vi "EnFlo_Tunnel_Setup.vi"() -> ()   [LabVIEW 2020]
uses:
  ADAM Controls/Update_scan_value.ctl
  ADAM Controls/Module_type_ADAM.ctl
  ADAM Controls/Function_ADAM.ctl
  ADAM Controls/Channel_State.ctl
  ADAM Controls/Calib_type_ADAM.ctl
  ADAM Controls/Address.ctl
  ADAM Controls/Ch_description_ADAM.ctl
panel:
  in  "Desired Lab Air Temp":dbl format="%.2f"
  out "Numerical Values":dbl[](array[numeric]) format="%.9f"
  out "Ch Description Array":T1[](array[typedef]) {"Duty" format="%016b"; "D" format="%#_5g"; "C" format="%#_5g"; "B" format="%#_5g"; "A" format="%#_5g"}
  in  "Traverse Origin X Offset (mm)":dbl min=0.0 max=20000.0
  in  "Show Heater Setup":bool
  in  "stop":bool
  in  "Desired Chilled Water Temp":dbl format="%.2f"
  out "Reference Anemometer":string
  in  "OK":bool
  in  "Wind Direction (Deg)":dbl format="%.2f"
  in  "Obstacle/Building":u16(ring) items=["1-500 DAPPLE low Res", "100mm Trench", "100x100 Cube", "100x100 pressure tapped cube", "100x100x200 Tall", "100x100x300 Tall", "100x100x400mm Tall", "110mm cube array 110mm spacing", "110mm cube array 55mm spacing", "12 WTs", "150*150*150mm cube", "16 blocks 55 x 55 x 110mm tall centre at x=12m", "16 buildings 250*500*125mm", "16 x 110mm cube array 110mm spacing", "20 buildings 500x250x125mm", "25 x 110mm cube array 110mm spacing", "25mm Trench in 1.4m Turntable", "4 buildings 750x500x125mm", "4 x 110mm cube array 110mm spacing", "400mm x 400mm Heated Mat centre 12m", "500x250x125 Block", "500x300mm Trees 100mm tall", "660mm x 3000mm Heated Mat centre 12m", "70x140x70bldgs 12x19rows 1x3h Building", "70x140x70bldgs 14x21row", "70x140x70bldgs 14x29 row", "9 x 110mm cube array 110mm spacing", "990mm x 3000mm Heated Mat centre 14m", "Array of 24 tanks dia 130mm height 88mm", "Blade 1", "Blade 2", "Building With Single Stack", "Building with Twin Stack", "Champs Elysees Source 1", "Champs Elysees Source 2", "Champs Elysees Source 3", "Complex - All buildings", "Complex - only 2 buildings", "Complex Array", "Concawe Actual Model 6 Cylinders", "DAPPLE Dome Centre", "DAPPLE Dome Centre with station", "DAPPLE high Res buildings at intersection", "DAPPLE low Res", "DAPPLE low Res with roof roughness", "DAPPLE low Res(model+B42-45 and obstacles in the west of the model)", "DAPPLE low Res(sampling at Mary  Rd  Model+B42-45)", "DAPPLE low Res(sampling at Mary  Rd with B38-41and A5)", "DAPPLE low Res(sampling at Mary  Rd without B38-41)", "DAPPLE low Res(sampling at Mary. Rd add A1-5)", "DYCE_London_110mm", "False Floor (table 4.17m x 0.9m  height 230mm)", "Forest at x=11003", "Group of 2 Tanks D=133mm upstream tank", "Group of 6 Tanks D=400mm no downstream tanks", "Group of 9 Tanks D=133mm Centre releasing 67mm roof heights", "Group of 9 Tanks D=400mm 3 downstream tanks", "HRModUrb SimpleC", "HRModUrb SimpleC with tall building", "HRModUrb SimpleV", "Headstart07 building", "Mesh Wool Disc Trees 220mm spacing", "Moditic_Bump", "Moditic_Bump_0-1385mm_200mm false floor", "Moditic_Bump_0-1385mm_200mm false floor No roughness", "Moditic_Bump_0-1385mm_200mm false floor with Array", "Moditic_Bump_0-1385mm_200mm false floor with Array_2", "Network Regular", "None", "Norway 1:300", "Norway 1:500", "ROSE (Bremen)", "Row_of_blocks_H=204_L=250mm", "S1_0Deg", "S1_45Deg", "S2_0Deg", "Sellafiield Site Model", "Sellafiield Site Model (Flat)", "Single Turbine II", "Single wind turbine (blade II) at X=10000 Y=0", "St Thomas Hospital - East Wing - Unclad", "St Thomas Hospital - East Wing - clad", "Storage Tank H=100  D=400mm", "Storage Tank H=100  D=400mm with 0 Deg Bund", "Storage Tank H=100  D=400mm with 45 Deg Bund", "Storage Tank H=100  D=400mm with Bund plus upstream tank", "Storage Tank H=100 D=500mmStorage Tank H=100  D=700mm", "Storage Tank H=89  D=133mm", "Storage Tank H=89  D=133mm with 0 Deg Bund", "Storage Tank H=89  D=133mm with 266mm Bund on turn table", "Storage Tank H=89  D=133mm with 45 Deg Bund", "Subfloor trench 285x285x3m", "Tree 171 mm - Dense", "Tree 171 mm - Porous", "Tree 91 mm - Dense", "Tree 91 mm - Porous", "Tree85mmRow - x=13000", "Two-Buildings Config", "Vehicle 1to20 - False Floor (table 4.17m x 0.9m  height 230mm)", "Vehicle 1to5 - False Floor (table 4.17m x 0.9m  height 230mm)", "WT Array1", "WT Array2", "WT Array21", "WT Array3", "WT Array4", "WT Array5", "WT Array6", "WT Array7", "WT x 2", "WT x 3", "WT x 4", "Edit Strings"]
  in  "Vorticity Generators":u16(ring) items=["5 Irwin spires 1.26m   X=50mm Y spacing 630mm", "5 Irwin spires 1.2m   X=50mm Y spacing 700mm", "Not Installed", "Offshore 13x TruncIrwin (H:600)  B(H:0):60  B(H:600):4  Yspace: 266  X:3925", "Offshore 13x TruncIrwin (H:600)  B(H:0):60  B(H:600):4  Yspace: 266  X:50", "Offshore 21x TruncIrwin (H:600)  B(H:0):60  B(H:600):4  Yspace: 167  X:50", "Offshore 5x TruncIrwin (H:1490)  B(H:0):150  B(H:1490):10  Yspace:660  X:50", "Offshore 5x TruncIrwin (H:1490)  B(H:0):150  B(H:700):10  Yspace:660  X:50", "Offshore 5x TruncIrwin (H:300)  B(H:0):150  B(H:300):10  Yspace:660  X:50", "Offshore 5x TruncIrwin (H:300)  B(H:0):30  B(H:300):2  Yspace:132  X:50", "Offshore 8x TruncIrwin (H:300)  B(H:0):150  B(H:300):10  Yspace:420  X:50", "Onshore 5xTruncNonIrwin (H:1490  B(H:0-120):250  B(H:192):177  B(H:1490):24)  YSpace:660 X:50", "Edit Strings"]
  in  "Side Wall Separation":u16(ring) items=["1.07m", "1.5m", "2.0m", "2.5m", "2.93m", "3m  from x=0.67 to x=10.67m", "3m  from x=0.67 to x=12.67m", "3m  from x=0.67 to x=18m", "3m  from x=0.67 to x=6.67m", "3m  from x=12 to x=18m", "3m  from x=2 to x=19m", "3m  from x=8 to x=18m", "No sidewalls installed", "Edit Strings"]
  in  "Roughness Height":u16(ring) items=["H=16mm  W=50mm Yspace=510mm Xspace=360mm Staggered", "H=20mm W=80mm YSpace=240mm  XSpace=240mm Staggered", "H=20mm W=80mm YSpace=240mm  XSpace=720mm Staggered", "no roughness elements (smooth)", "Edit Strings"]
  # "Boundary Layer Generation setup"
  # "This value should be zero if working in tunnel coordinates  (X=0 at start of working section)"
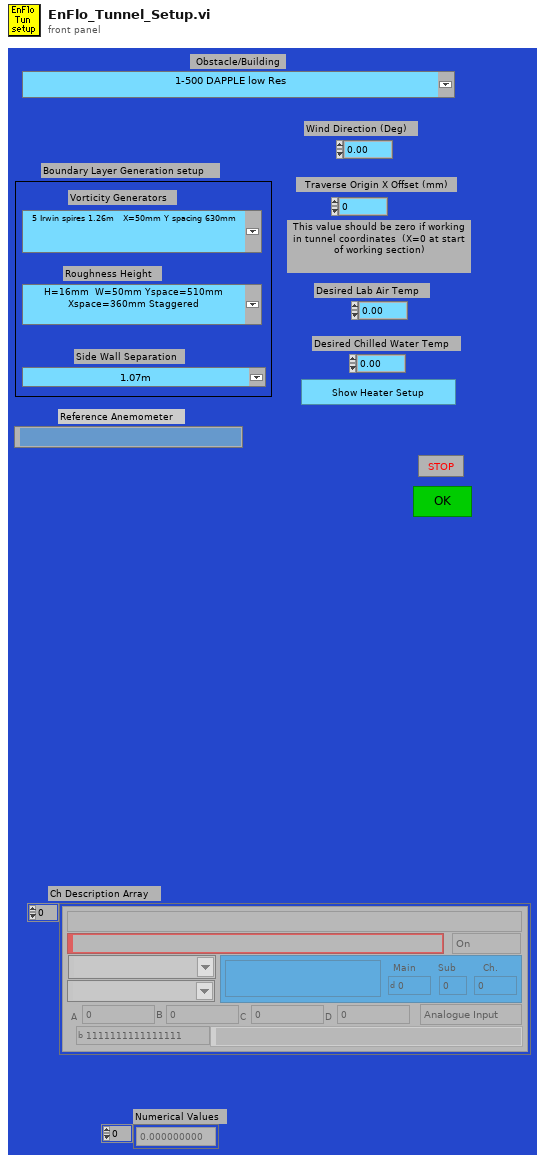
[diagram p1: front panel]
types:
  T1 = typedef "Ch_description_ADAM.ctl" = cluster{"Ch Name":string, "Type":T2, "Function":T3, "Ch State":T4, "Calibration type":T5, "A":dbl, "B":dbl, "C":dbl, "D":dbl, "Comments":string, "Address":T6, "String":string, "Duty":u16}
  T2 = typedef "Module_type_ADAM.ctl" = string
  T3 = typedef "Function_ADAM.ctl" = enum16{"Analogue Input", "Digital Input", "Event counter", "Event rate", "Analogue Output", "Digital Output", "Relay Output"}
  T4 = typedef "Channel_State.ctl" = enum16{"On", "Off", "Always On", "Always Off"}
  T5 = typedef "Calib_type_ADAM.ctl" = string
  T6 = typedef "Address.ctl" = cluster{"Main":i32, "Ch.":i32, "Sub":i32, "Port Name":string}
  T7 = typedef "Update_scan_value.ctl" = cluster{"Channel Name":string, "New Value":dbl}
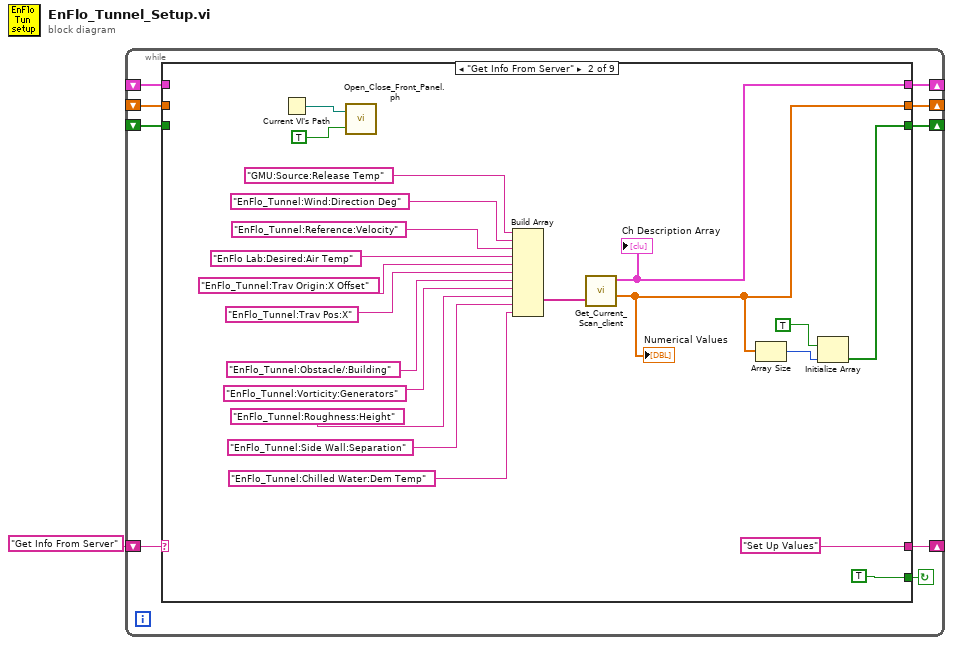
[diagram p0: block diagram]
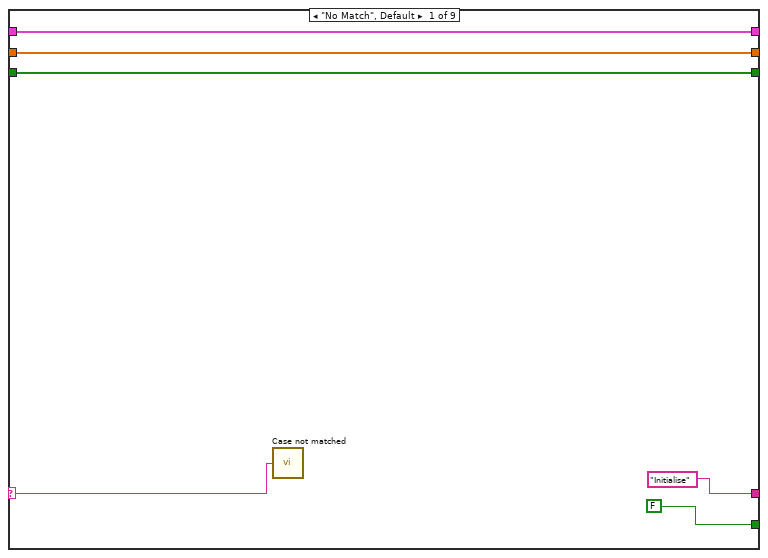
[diagram p2: hidden frame]
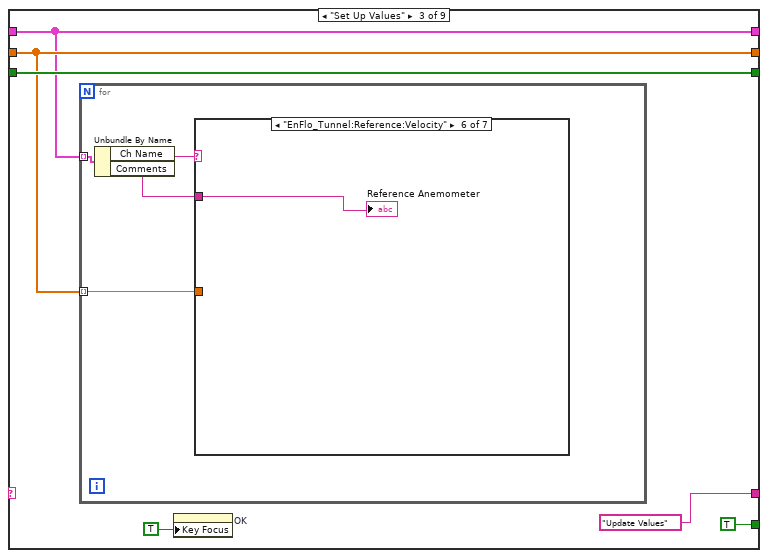
[diagram p3: hidden frame]
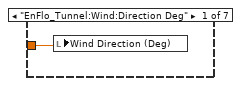
[diagram p4: hidden frame]
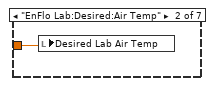
[diagram p5: hidden frame]
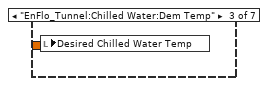
[diagram p6: hidden frame]
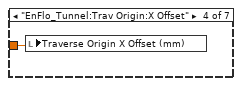
[diagram p7: hidden frame]
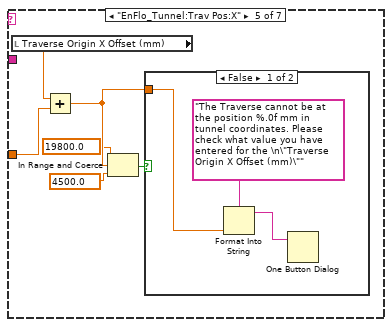
[diagram p8: hidden frame]
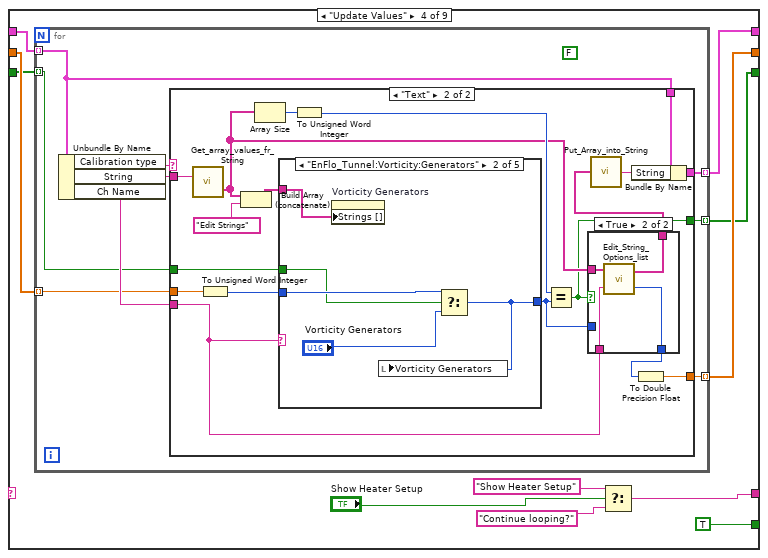
[diagram p11: hidden frame]
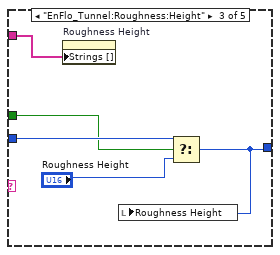
[diagram p15: hidden frame]
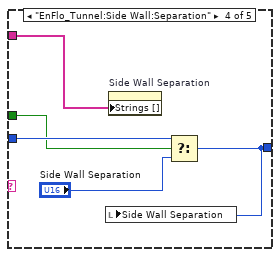
[diagram p16: hidden frame]
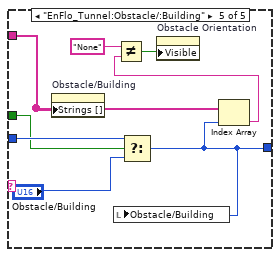
[diagram p17: hidden frame]
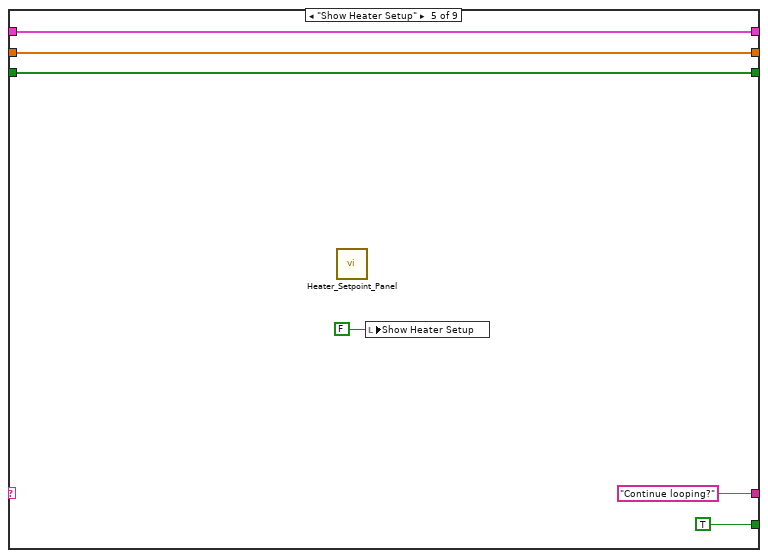
[diagram p18: hidden frame]
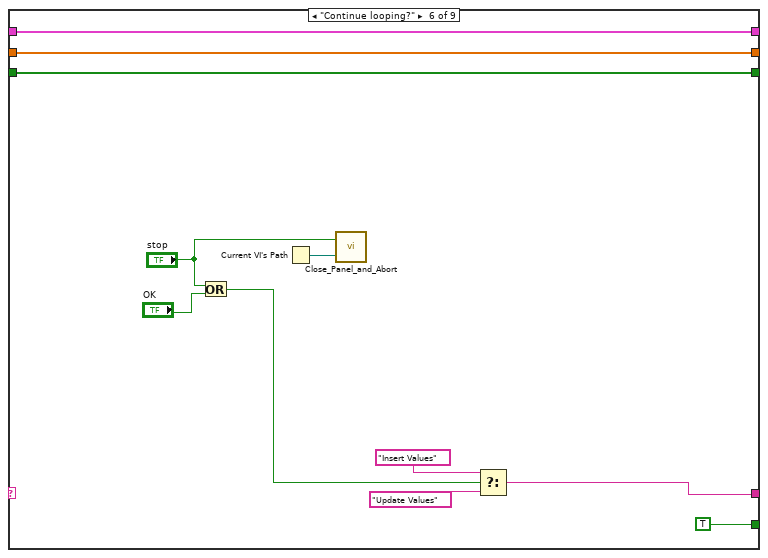
[diagram p19: hidden frame]
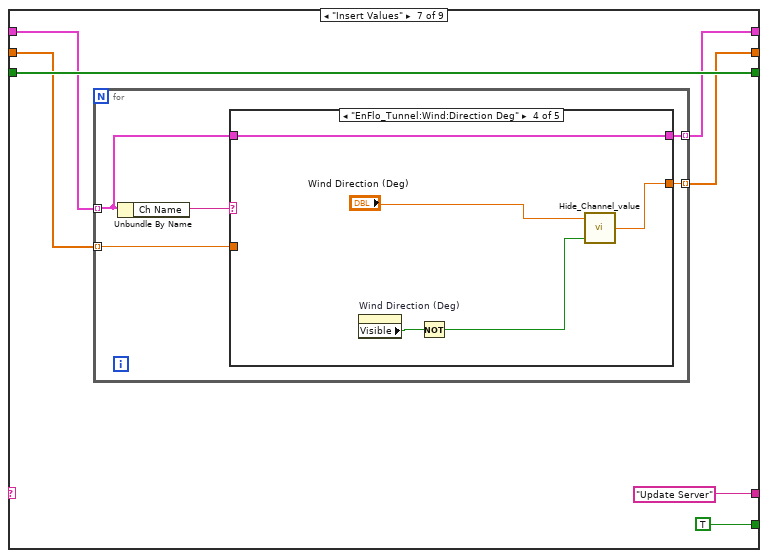
[diagram p20: hidden frame]
diagram:
  n1 = while {
    shift-left: _ -> [w2]
    shift-right: [w3] -> _
    shift-left: _ -> [w4]
    shift-right: [w6] -> _
    shift-left: _ -> [w5]
    shift-right: [w7] -> _
    shift-left: "Get Info From Server" -> [w8]
    shift-right: [w9] -> _
    stop <- w10 continue-if-true
    n2 = case shown="\"Get Info From Server\"" w8 {
      selector: w8 -> [w11 _ _ _ _ _ _ _ _]
      tunnel: [FALSE TRUE TRUE ("T button?") TRUE ("T button?") TRUE ("T button?") TRUE ("T button?") TRUE ("T button?") TRUE ("T button?") FALSE ("T button?")] -> w10
      tunnel: ["Initialise" "Set Up Values" "Update Values" w66 "Continue looping?" w140 "Update Server" "Add comments etc" "End"] -> w9
      tunnel: [w14 w28 w39 w70 w138 w149 w150 w182 w226] -> w7
      tunnel: [w13 w27 w40 w68 w137 w148 w153 w181 w225] -> w6
      tunnel: w5 -> [w14 _ w39 w71 w138 w149 w151 w182 w226]
      tunnel: w4 -> [w13 _ w40 w69 w137 w148 w152 w181 w225]
      tunnel: [w12 w24 w42 w62 w134 w146 w155 w180 w223] -> w3
      tunnel: w2 -> [w12 _ w42 w63 w134 w146 w155 w180 w223]
      frame "No Match", Default {
        n3 = call "Case not matched.vi"("Case Name not Matched"=w11) -> ()
      }
      frame "Get Info From Server" {
        n4 = Current VI's Path() -> (path=w22:path)
        n5 = call "Open_Close_Front_Panel.ph.vi"("Front Panel Window:Open"=TRUE, "VI path"=w22) -> ()  [unwired: 2 out]
        n6 = Build Array("GMU:Source:Release Temp", "EnFlo_Tunnel:Wind:Direction Deg", "EnFlo_Tunnel:Reference:Velocity", "EnFlo Lab:Desired:Air Temp", "EnFlo_Tunnel:Trav Origin:X Offset", "EnFlo_Tunnel:Trav Pos:X", "EnFlo_Tunnel:Obstacle/:Building", "EnFlo_Tunnel:Vorticity:Generators", "EnFlo_Tunnel:Roughness:Height", "EnFlo_Tunnel:Side Wall:Separation", "EnFlo_Tunnel:Chilled Water:Dem Temp") -> (w35:string[])
        n7 = call "Get_Current_Scan_client.vi"("multipleChannels"=w35) -> ("Ch Description Array"=w28:T1[], "Numerical Values"=w27:dbl[])  [unwired: 2 in, 1 out]
        "Ch Description Array" <- w28
        "Numerical Values" <- w27
        n8 = Array Size(array=w27) -> (size(s)=w26:i32)
        n9 = Initialize Array(TRUE, w26) -> (w24:bool[])
      }
      frame "Set Up Values" {
        n10 = for {
          tunnel: w40 -> [w47] mode=indexing
          tunnel: w39 -> [w46] mode=indexing
          n11 = Unbundle By Name(w46) -> ("Ch Name"=w45:string, "Comments"=w44:string)
          n12 = case shown="\"EnFlo_Tunnel:Reference:Velocity\"" w45 {
            tunnel: w47 -> [w48 w49 w50 w51 w56 _ _]
            tunnel: w44 -> [_ _ _ _ _ w61 _]
            frame "EnFlo_Tunnel:Wind:Direction Deg" {
              n13 = local write "Wind Direction (Deg)"(w48) -> ()
            }
            frame "EnFlo Lab:Desired:Air Temp" {
              n14 = local write "Desired Lab Air Temp"(w49) -> ()
            }
            frame "EnFlo_Tunnel:Chilled Water:Dem Temp" {
              n15 = local write "Desired Chilled Water Temp"(w50) -> ()
            }
            frame "EnFlo_Tunnel:Trav Origin:X Offset" {
              n16 = local write "Traverse Origin X Offset (mm)"(w51) -> ()
            }
            frame "EnFlo_Tunnel:Trav Pos:X" {
              n17 = local read "Traverse Origin X Offset (mm)"() -> (w57:dbl)
              n18 = Add(x=w57, y=w56) -> (x+y=w55:dbl)
              n19 = In Range and Coerce(upper limit=19800.0 ("y"), x=w55, lower limit=4500.0 ("y")) -> (In Range?=w52:bool)  [unwired: 1 out]
              n20 = case shown="False" w52 {
                tunnel: w55 -> [w60 _]
                frame False {
                  n21 = Format Into String(format string="The Traverse cannot be at the position %.0f mm in tunnel coordinates. Please check what value you have entered for the \n\"Traverse Origin X Offset (mm)\"" ("Format String"), w60) -> (resulting string=w58:string)  [unwired: 2 in, 1 out]
                  n22 = One Button Dialog(message=w58) -> ()  [unwired: 2 out]
                }
                frame True {
                }
              }
            }
            frame "EnFlo_Tunnel:Reference:Velocity" {
              "Reference Anemometer" <- w61
            }
            frame "No Match", Default {
            }
          }
        }
        n23 = property on="OK" class="Bool"("Key Focus"=TRUE ("Write Attribute")) -> ()  [unwired: 2 in, 2 out]
      }
      frame "Update Values" {
        n24 = for {
          tunnel: w71 -> [w78] mode=indexing
          tunnel: [w77] -> w70 mode=indexing
          tunnel: w69 -> [w76] mode=indexing
          tunnel: [w75] -> w68 mode=indexing
          tunnel: w63 -> [w74] mode=indexing
          tunnel: [w73] -> w62 mode=indexing
          (unwired) FALSE
          n25 = Unbundle By Name(w78) -> ("Calibration type"=w81:T5, "String"=w80:string, "Ch Name"=w79:string)
          n26 = case shown="\"Text\"" w81 {
            tunnel: w80 -> [_ w102]
            tunnel: w79 -> [_ w92]
            tunnel: w78 -> [w84 w96]
            tunnel: [w84 w95] -> w77
            tunnel: w76 -> [w83 w94]
            tunnel: [w83 w93] -> w75
            tunnel: w74 -> [w82 w91]
            tunnel: [w82 w85] -> w73
            frame "Raw", Default {
            }
            frame "Text" {
              n27 = call "Get_array_values_fr_String.vi"("String Value"=w102) -> ("String array"=w90:string[])  [unwired: 1 out]
              n28 = To Unsigned Word Integer(number=w94) -> (unsigned 16bit integer=w100:u16)
              n29 = Build Array (concatenate)(w90, "Edit Strings") -> (w89:string[])
              n30 = Array Size(array=w90) -> (size(s)=w101:i32)
              n31 = case shown="\"EnFlo_Tunnel:Vorticity:Generators\"" w92 {
                tunnel: [w109 w112 w117 w121 w129] -> w86
                tunnel: w89 -> [_ w111 w116 w122 w131]
                tunnel: w100 -> [w109 w114 w119 w124 w132]
                tunnel: w91 -> [_ w110 w115 w120 w125]
                frame "No match", Default {
                }
                frame "EnFlo_Tunnel:Vorticity:Generators" {
                  n32 = property on="Vorticity Generators" class="Ring (strict)"("Strings []"=w111) -> ()  [unwired: 2 in, 2 out]
                  n33 = Select(t=w114, s=w110, f="Vorticity Generators") -> (s? t:f=w112:u16)
                  n34 = local write "Vorticity Generators"(w112) -> ()
                }
                frame "EnFlo_Tunnel:Roughness:Height" {
                  n35 = property on="Roughness Height" class="Ring (strict)"("Strings []"=w116) -> ()  [unwired: 2 in, 2 out]
                  n36 = Select(t=w119, s=w115, f="Roughness Height") -> (s? t:f=w117:u16)
                  n37 = local write "Roughness Height"(w117) -> ()
                }
                frame "EnFlo_Tunnel:Side Wall:Separation" {
                  n38 = property on="Side Wall Separation" class="Ring (strict)"("Strings []"=w122) -> ()  [unwired: 2 in, 2 out]
                  n39 = Select(t=w124, s=w120, f="Side Wall Separation") -> (s? t:f=w121:u16)
                  n40 = local write "Side Wall Separation"(w121) -> ()
                }
                frame "EnFlo_Tunnel:Obstacle/:Building" {
                  n41 = property on="Obstacle/Building" class="Ring (strict)"("Strings []"=w131) -> ()  [unwired: 2 in, 2 out]
                  n42 = Select(t=w132, s=w125, f="Obstacle/Building") -> (s? t:f=w129:u16)
                  n43 = local write "Obstacle/Building"(w129) -> ()
                  n44 = Index Array(array=w131, index=w129) -> (element=w126:string)
                  n45 = Not Equal?(x="None", y=w126) -> (x != y?=w127:bool)
                  n46 = property on="Obstacle Orientation" class="DigNum (strict)"("Visible"=w127) -> ()  [unwired: 2 in, 2 out]
                }
              }
              n47 = To Unsigned Word Integer(number=w101) -> (unsigned 16bit integer=w99:u16)
              n48 = Equal?(x=w99, y=w86) -> (x = y?=w85:bool)
              n49 = case shown="True" w85 {
                tunnel: w90 -> [w104 w108]
                tunnel: w92 -> [_ w107]
                tunnel: [w104 w106] -> w97
                tunnel: [w103 w105] -> w87
                tunnel: w86 -> [w103 _]
                frame False {
                }
                frame True {
                  n50 = call "Edit_String_Options_list.vi"("Channel Name"=w107, "String array"=w108) -> ("New Selection Index"=w105:i32, "String array Out"=w106:string[])
                }
              }
              n51 = call "Put_Array_into_String.vi"("String array"=w97) -> ("String Value"=w98:string)
              n52 = Bundle By Name(cluster=w96, "String"=w98) -> (w95:T1)
              n53 = To Double Precision Float(number=w87) -> (double precision float=w93:dbl)
            }
          }
        }
        n54 = Select(t="Show Heater Setup", s="Show Heater Setup", f="Continue looping?") -> (s? t:f=w66:string)
      }
      frame "Show Heater Setup" {
        n55 = call "Heater_Setpoint_Panel.vi"() -> ()  [unwired: 1 out]
        n56 = local write "Show Heater Setup"(FALSE ("Show Inlet heater Setup")) -> ()
      }
      frame "Continue looping?" {
        n57 = Or(x="stop", y="OK") -> (x .or. y?=w143:bool)
        n58 = Current VI's Path() -> (path=w145:path)
        n59 = call "Close_Panel_and_Abort.vi"("Vi path"=w145, "stop"="stop") -> ()  [unwired: 1 out]
        n60 = Select(t="Insert Values", s=w143, f="Update Values") -> (s? t:f=w140:string)
      }
      frame "Insert Values" {
        n61 = for {
          tunnel: w151 -> [w158] mode=indexing
          tunnel: w152 -> [w160] mode=indexing
          tunnel: [w159] -> w153 mode=indexing
          tunnel: [w157] -> w150 mode=indexing
          n62 = Unbundle By Name(w158) -> ("Ch Name"=w161:string)
          n63 = case shown="\"EnFlo_Tunnel:Wind:Direction Deg\"" w161 {
            tunnel: w160 -> [_ _ _ _ w174]
            tunnel: ["Desired Lab Air Temp" "Desired Chilled Water Temp" "Traverse Origin X Offset (mm)" w169 w174] -> w159
            tunnel: w158 -> [w163 w165 w166 w168 w173]
            tunnel: [w163 w165 w166 w168 w173] -> w157
            frame "EnFlo Lab:Desired:Air Temp" {
            }
            frame "EnFlo_Tunnel:Chilled Water:Dem Temp" {
            }
            frame "EnFlo_Tunnel:Trav Origin:X Offset" {
            }
            frame "EnFlo_Tunnel:Wind:Direction Deg" {
              n64 = property on="Wind Direction (Deg)" class="DigNum (strict)"() -> ("Visible"=w172:bool)  [unwired: 2 in, 2 out]
              n65 = Not(x=w172) -> (.not. x?=w171:bool)
              n66 = call "Hide_Channel_value.vi"("Hide Values"=w171, "Value In"="Wind Direction (Deg)") -> ("Value Out"=w169:dbl)  [unwired: 1 in]
            }
            frame "No Match", Default {
            }
          }
        }
      }
      frame "Update Server" {
        w177 = T7 {"Channel Name"="", "New Value"=0.0} ("Update Scan Value Cluster")
        n67 = Index Array(array=w182, index=0 ("Index")) -> (element=w193:T1)
        n68 = local read "Ch Description Array"() -> (w179:T1[])
        n69 = local read "Numerical Values"() -> (w178:dbl[])
        n70 = Initialize Array(w193, 0 ("Dimension Size")) -> (w191:T1[])
        n71 = Initialize Array(w177, 0 ("Dimension Size")) -> (w186:T7[])
        n72 = for {
          shift-right: [w206] -> w188
          shift-left: w191 -> [w207]
          tunnel: w182 -> [w197] mode=indexing
          shift-right: [w205] -> w183
          shift-left: w186 -> [w204]
          tunnel: w181 -> [w199] mode=indexing
          tunnel: w179 -> [w198] mode=indexing
          tunnel: w178 -> [w202] mode=indexing
          tunnel: w177 -> [w200]
          n73 = Equal?(x=w197, y=w198) -> (x = y?=w203:bool)
          n74 = Equal?(x=w199, y=w202) -> (x = y?=w201:bool)
          n75 = case shown="False" w201 {
            tunnel: w204 -> [w214 w215]
            tunnel: [w213 w215] -> w205
            tunnel: w200 -> [w212 _]
            tunnel: w199 -> [w211 _]
            tunnel: w197 -> [w210 _]
            frame False {
              n76 = Unbundle By Name(w210) -> ("Ch Name"=w209:string)
              n77 = Bundle By Name(cluster=w212, "Channel Name"=w209, "New Value"=w211) -> (w208:T7)
              n78 = Build Array (concatenate)(w214, w208) -> (w213:T7[])
            }
            frame True {
            }
          }
          n79 = case shown="False" w203 {
            tunnel: w207 -> [w218 w219]
            tunnel: w197 -> [w217 _]
            tunnel: [w216 w219] -> w206
            frame False {
              n80 = Build Array (concatenate)(w218, w217) -> (w216:T1[])
            }
            frame True {
            }
          }
        }
        n81 = Array Size(array=w188) -> (size(s)=w190:i32)
        n82 = Array Size(array=w183) -> (size(s)=w184:i32)
        n83 = Greater Than 0?(x=w190) -> (x > 0?=w189:bool)
        n84 = Greater Than 0?(x=w184) -> (x > 0?=w185:bool)
        n85 = case shown="True" w189 {
          tunnel: w188 -> [_ w196]
          frame False {
          }
          frame True {
            n86 = call "Update_Ch_Discription_client.vi"("Channels to update In"=w196) -> ()  [unwired: 1 out]
          }
        }
        n87 = case shown="True" w185 {
          tunnel: w183 -> [_ w195]
          frame False {
          }
          frame True {
            n88 = call "Update_Current_Value_client.vi"("Update array in"=w195) -> ()  [unwired: 1 in]
          }
        }
      }
      frame "Add comments etc" {
        n89 = Current VI's Path() -> (path=w220:path)
        n90 = call "Open_Close_Front_Panel.ph.vi"("Front Panel Window:Open"=FALSE, "VI path"=w220) -> ()  [unwired: 2 out]
      }
    }
  }
